vi "MATBuild.vi"(6 "Class in":T2(ring), 7 "byte order":T1(ring), 9 "Cluster":T3, 10 "Dimensions":i32[](array[numeric]), 11 "Name":string) -> (3 "String Out":string)   [LabVIEW 2022 SP3]
uses:
  miDataType.ctl
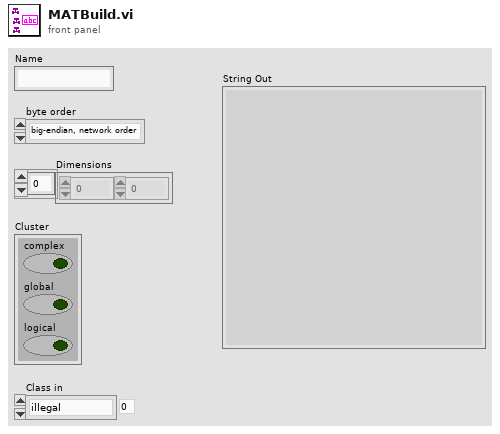
[diagram p1: front panel]
types:
  T1 = enum16{"big-endian, network order", "native, host order", "little-endian"}
  T2 = enum16{"illegal", "Cell array", "Structure", "Object", "Character Array", "Sparse Array", "Double Array", "Single Array", "i8", "u8", "i16", "u16", "i32", "u32", "i64", "u64"}
  T3 = cluster{"complex":bool, "global":bool, "logical":bool}
  T4 = typedef "miDataType.ctl" = enum16{"illegal", "miINT8", "miUINT8", "miINT16", "miUINT16", "miINT32", "miUINT32", "miSINGLE", "--", "miDOUBLE", "---", "----", "miINT64", "miUINT64", "miMATRIX", "miCOMPRESSED", "miUTF8", "miUTF16", "miUTF32", "udefined"}
  T5 = cluster{"Data Type":T4, "# bytes":u32, "data":string}
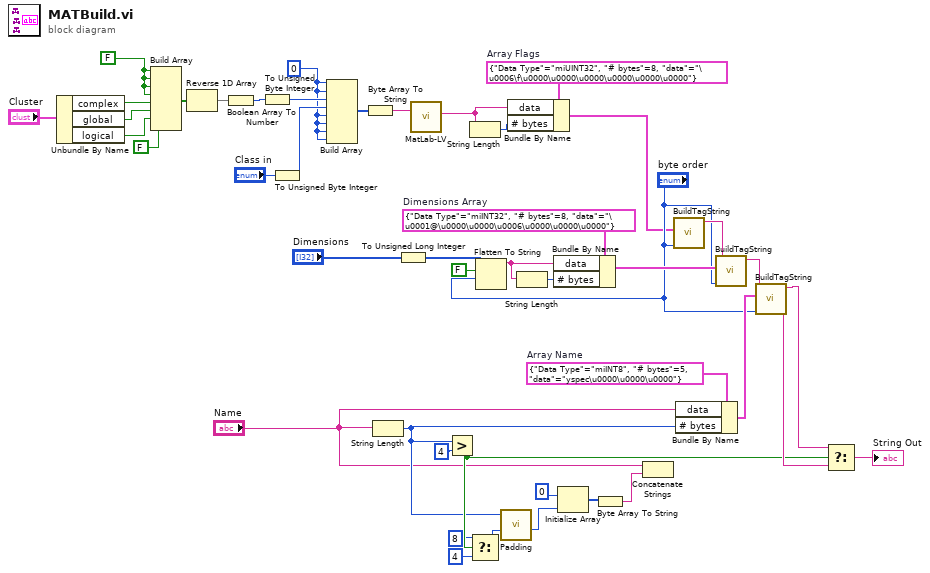
[diagram p0: block diagram]
diagram:
  w20 = u8 0
  w30 = FALSE
  w33 = T5 {"Data Type"=enum."miINT8", "# bytes"=5, "data"="yspec\u0000\u0000\u0000"}  # Array Name
  w43 = T5 {"Data Type"=enum."miINT32", "# bytes"=8, "data"="\u0001@\u0000\u0000\u0006\u0000\u0000\u0000"}  # Dimensions Array
  w15 = T5 {"Data Type"=enum."miUINT32", "# bytes"=8, "data"="\u0006\f\u0000\u0000\u0000\u0000\u0000\u0000"}  # Array Flags
  n1 = Unbundle By Name("Cluster") -> ("complex"=w29:bool, "global"=w28:bool, "logical"=w27:bool)
  n2 = Build Array(w30, w30, w30, w30, w29, w28, w27, FALSE) -> (w25:bool[])
  n3 = Reverse 1D Array(array=w25) -> (reversed array=w16:bool[])
  n4 = Boolean Array To Number(Boolean array=w16) -> (number=w24:u32)
  n5 = To Unsigned Byte Integer(number=w24) -> (unsigned 8bit integer=w22:u8)
  n6 = To Unsigned Byte Integer(number="Class in") -> (unsigned 8bit integer=w21:u8)
  n7 = Build Array(w20, w20, w22, w21, w20, w20, w20, w20) -> (w18:u8[])
  n8 = Byte Array To String(unsigned byte array=w18) -> (string=w17:string)
  n9 = String Length(string="Name") -> (length=w4:i32)
  n10 = To Unsigned Long Integer(number="Dimensions") -> (unsigned 32bit integer=w44:u32[])
  n11 = call "MatLab-LV.vi"("data in"=w17) -> ("data out"=w13:string)  [unwired: 10 in]
  n12 = Greater?(x=w4, y=4) -> (0:w9:bool)
  n13 = String Length(string=w13) -> (length=w14:i32)
  n14 = Select(t=8 ("y"), s=w9, f=4 ("y")) -> (s? t:f=w6:i32)
  n15 = Flatten To String(anything=w44, prepend array or string size? (T)=FALSE ("data includes array or string size? (T)"), byte order (0:big-endian, network order)="byte order") -> (data string=w42:string)  [unwired: 1 in, 2 out]
  n16 = call "Padding.vi"("size"=w6, "bytes in"=w4) -> ("padding"=w37:i32)  [unwired: 8 in, 1 out]
  n17 = Bundle By Name(cluster=w15, "data"=w13, "# bytes"=w14) -> (w5:T5)
  n18 = String Length(string=w42) -> (length=w41:i32)
  n19 = Bundle By Name(cluster=w43, "data"=w42, "# bytes"=w41) -> (w39:T5)
  n20 = Initialize Array(u8 0 ("element"), w37) -> (w35:u8[])
  n21 = Byte Array To String(unsigned byte array=w35) -> (string=w34:string)
  n22 = Concatenate Strings("Name", w34) -> ()  [unwired: 1 out]
  n23 = call "BuildTagString.vi"("byte order"="byte order", "Tag"=w5) -> ("String Out"=w40:string)  [unwired: 8 in, 1 out]
  n24 = Bundle By Name(cluster=w33, "data"="Name", "# bytes"=w4) -> (w32:T5)
  n25 = call "BuildTagString.vi"("byte order"="byte order", "Tag"=w39, "String In"=w40) -> ("String Out"=w38:string)  [unwired: 7 in, 1 out]
  n26 = call "BuildTagString.vi"("byte order"="byte order", "Tag"=w32, "String In"=w38) -> ("Compressed String Out"=w10:string, "String Out"=w11:string)  [unwired: 7 in]
  n27 = Select(t=w11, s=w9, f=w10) -> (s? t:f=→"String Out":string)
